vi "temp_FlpLib AlphaBetaToABC_PowInv.vi"(0 "alpha":sgl format="%#_32g", 5 "beta":sgl format="%#_32g") -> (4 "A":sgl format="%#_32g", 6 "B":sgl, 8 "C":sgl)   [LabVIEW 2016]
uses:
  <userlib>/_NI FLP Library/FPGA/outsideSCTL/FlpLib Multiply Shared Instance 0.vi
  <userlib>/_NI FLP Library/FPGA/outsideSCTL/FlpLib Subtract Shared Instance 0.vi
  <userlib>/_NI FLP Library/FPGA/outsideSCTL/FlpLib Add Shared Instance 0.vi
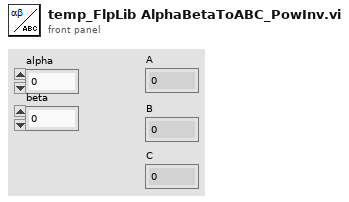
[diagram p1: front panel]
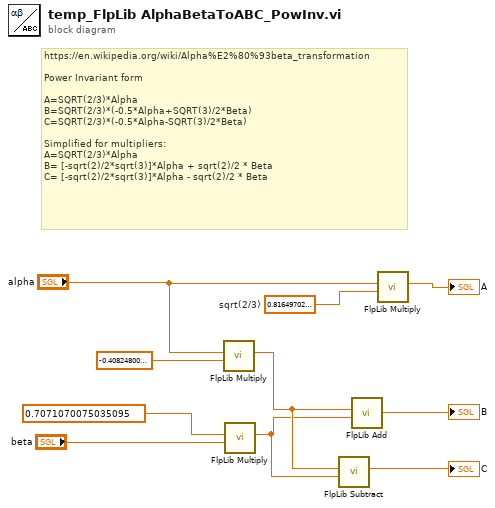
[diagram p0: block diagram]
diagram:
  w6 = sgl 0.816497  # sqrt(2/3)
  # "https://en.wikipedia.org/wiki/Alpha%E2%80%93beta_transformation\n\nPower Invariant form\n\nA=SQRT(2/3)*Alpha\nB=SQRT(2/3)*(-0.5*Alpha+SQRT(3)/2*Beta)\nC=SQRT(2/3)*(-0.5*Alpha-SQRT(3)/2*Beta)\n\nSimplified for multipliers:\nA=SQRT(2/3)*Alpha\nB= [-sqrt(2)/2*sqrt(3)]*Alpha + sqrt(2)/2 * Beta\nC= [-sqrt(2)/2*sqrt(3)]*Alpha - sqrt(2)/2 * Beta"
  n1 = call-poly <userlib>:"FlpLib Multiply.vi"("y"=sgl -0.408248, "x"="alpha") -> ("x*y"=w3:sgl)  [unwired: 5 in]
  n2 = call-poly <userlib>:"FlpLib Multiply.vi"("y"="beta", "x"=sgl 0.707107 ("beta")) -> ("x*y"=w2:sgl)  [unwired: 5 in]
  n3 = call-poly <userlib>:"FlpLib Subtract.vi"("y"=w2, "x"=w3) -> ("x-y"=→"C":sgl)  [unwired: 5 in]
  n4 = call-poly <userlib>:"FlpLib Add.vi"("y"=w2, "x"=w3) -> ("x+y"=→"B":sgl)  [unwired: 5 in]
  n5 = call-poly <userlib>:"FlpLib Multiply.vi"("y"=w6, "x"="alpha") -> ("x*y"=→"A":sgl)  [unwired: 5 in]
